vi "Read Data.vi"(8 "error in (no error)":errorcluster, 10 "Count":i32=-1, 11 "Stream in":refnum<class "Stream.lvclass">) -> (0 "error out":errorcluster, 2 "Data":string, 3 "Stream out":refnum<class "Stream.lvclass">)   [LabVIEW 2020, in "Stream.lvlib" / "Stream.lvclass"]
doc: "Reads the specified amount of data from the stream. Special count values are:\n\n-1: Read all available data within timeout or end of stream\n0: Read length prepended message\n\nReading a length prepended message first reads 4 bytes from the stream to get a 4 byte length and then reads that many bytes as the data. This is useful for reading variable length data as long as the length was also prepended to the data that was written."
uses:
  Stream.lvclass
  Data Direction.ctl
  Stream.lvlib
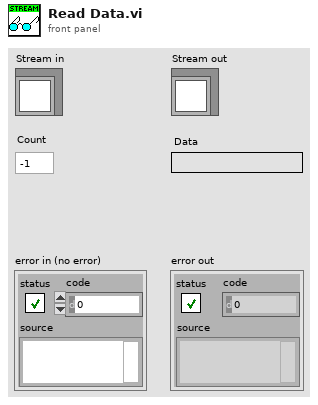
[diagram p1: front panel]
types:
  T1 = typedef "Stream.lvlib/Data Direction.ctl" = enum16{"Incoming", "Outgoing"}
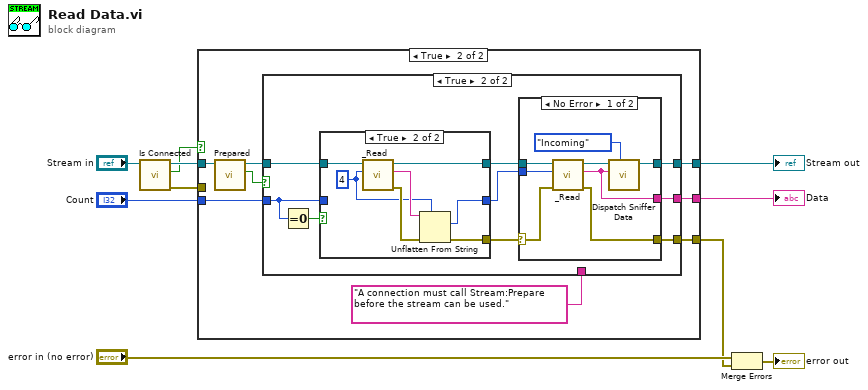
[diagram p0: block diagram]
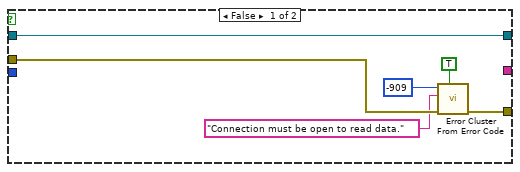
[diagram p2: hidden frame]
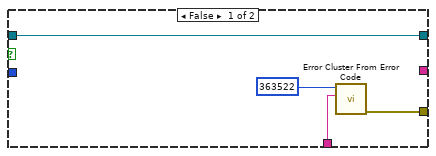
[diagram p3: hidden frame]
diagram:
  n1 = call-dynamic "Is Connected.vi"("Stream in"="Stream in") -> ("error out"=w1:errorcluster, "Connected"=w2:bool, "Stream out"=w3:refnum<class "Stream.lvclass">)  [unwired: 8 in]
  n2 = case shown="True" w2 {
    tunnel: [w16 w21] -> w8
    tunnel: [w15 w20] -> w6
    tunnel: [_ w19] -> w5
    tunnel: "Count" -> [_ w18]
    tunnel: w3 -> [w16 w17]
    tunnel: w1 -> [w12 _]
    frame False {
      n3 = call <vilib>:"Error Cluster From Error Code.vi"("show call chain? (False)"=TRUE, "error in (no error)"=w12, "error message (\"\")"="Connection must be open to read data.", "error code (0)"=-909) -> ("error out"=w15:errorcluster)  [unwired: 5 in]
    }
    frame True {
      n4 = call "Prepared.vi"("Stream in"=w17) -> ("Prepared"=w23:bool, "Stream out"=w24:refnum<class "Stream.lvclass">)  [unwired: 8 in, 1 out]
      n5 = case shown="True" w23 {
        tunnel: w18 -> [_ w32]
        tunnel: [w27 w37] -> w20
        tunnel: [_ w35] -> w19
        tunnel: [w28 w36] -> w21
        tunnel: w24 -> [w28 w34]
        tunnel: "A connection must call Stream:Prepare before the stream can be used." ("error message (\"\")") -> [w25 _]
        frame False {
          n6 = call <vilib>:"Error Cluster From Error Code.vi"("error message (\"\")"=w25, "error code (0)"=363522) -> ("error out"=w27:errorcluster)  [unwired: 7 in]
        }
        frame True {
          n7 = Equal To 0?(x=w32) -> (x = 0?=w33:bool)
          n8 = case shown="True" w33 {
            tunnel: w34 -> [w48 w55]
            tunnel: w32 -> [w49 _]
            tunnel: [w49 w51] -> w31
            tunnel: [w48 w54] -> w30
            tunnel: [_ w50] -> w29
            frame False {
            }
            frame True {
              w52 = 4 ("Count")
              n9 = call-dynamic "_Read.vi"("Count"=w52, "Stream in"=w55) -> ("error out"=w56:errorcluster, "Data"=w53:string, "Stream out"=w54:refnum<class "Stream.lvclass">)  [unwired: 7 in]
              n10 = Unflatten From String(type=w52, binary string=w53, error in (no error)=w56) -> (value=w51:i32, error out=w50:errorcluster)  [unwired: 2 in, 1 out]
            }
          }
          n11 = case shown="No Error" w29 {
            selector: w29 -> [w38 w46]
            tunnel: [w45 w46] -> w37
            tunnel: [w42 w47] -> w36
            tunnel: [w41 _] -> w35
            tunnel: w31 -> [w40 _]
            tunnel: w30 -> [w39 w47]
            frame No Error {
              n12 = call-dynamic "_Read.vi"("error in (no error)"=w38, "Count"=w40, "Stream in"=w39) -> ("error out"=w45:errorcluster, "Data"=w41:string, "Stream out"=w44:refnum<class "Stream.lvclass">)  [unwired: 6 in]
              n13 = call "Dispatch Sniffer Data.vi"("Data Direction"=Data_Direction."Incoming", "Data"=w41, "Stream in"=w44) -> ("Stream out"=w42:refnum<class "Stream.lvclass">)  [unwired: 7 in, 1 out]
            }
            frame Error {
            }
          }
        }
      }
    }
  }
  "Stream out" <- w8
  "Data" <- w5
  n14 = Merge Errors("error in (no error)", w6) -> (→"error out":errorcluster)
